vi "FindNodeAtIndex.vi"(8 "ClickIndex":u32=26, 10 "XML with IDs":string="<Sequential ID-O-3=\"\">\n      <Sequential ID-C-1=\"\">\n      </Sequential ID-C-1=\"\">\n      <Drive ID-C-2=\"\"/>\n</Sequential>", 11 "XML In":string="<Sequential>\n      <Sequential>\n      </Sequential>\n      <Drive/>\n</Sequential>") -> (0 "Insert as child not sibling":bool, 1 "Node Name":string="Drive", 3 "Node ID":string)   [LabVIEW 2019]
uses:
  <vilib>/regexp/Match Regular Expression.xnode
panel:
  out "submatch 1":string
  out "String":string
  out "submatch 2":string
  out "Line":i32
  out "Text.Selection:Start":u32=66
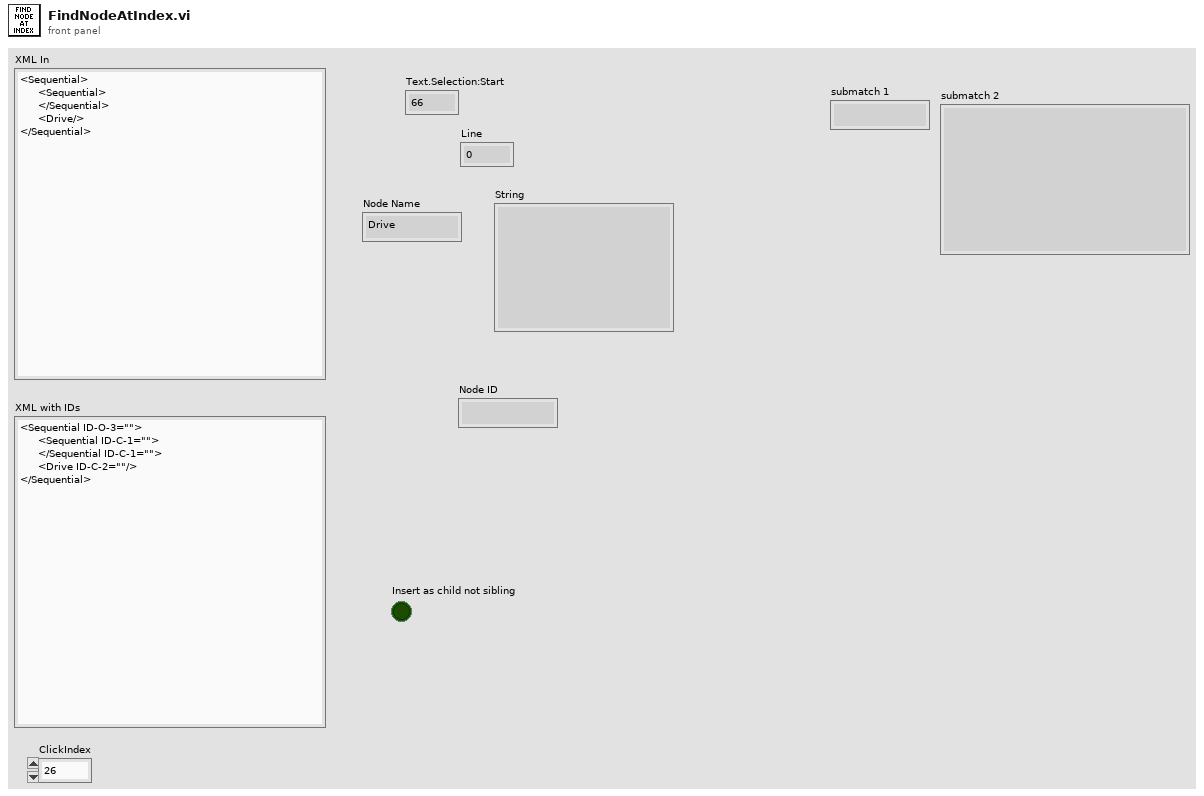
[diagram p1: front panel]
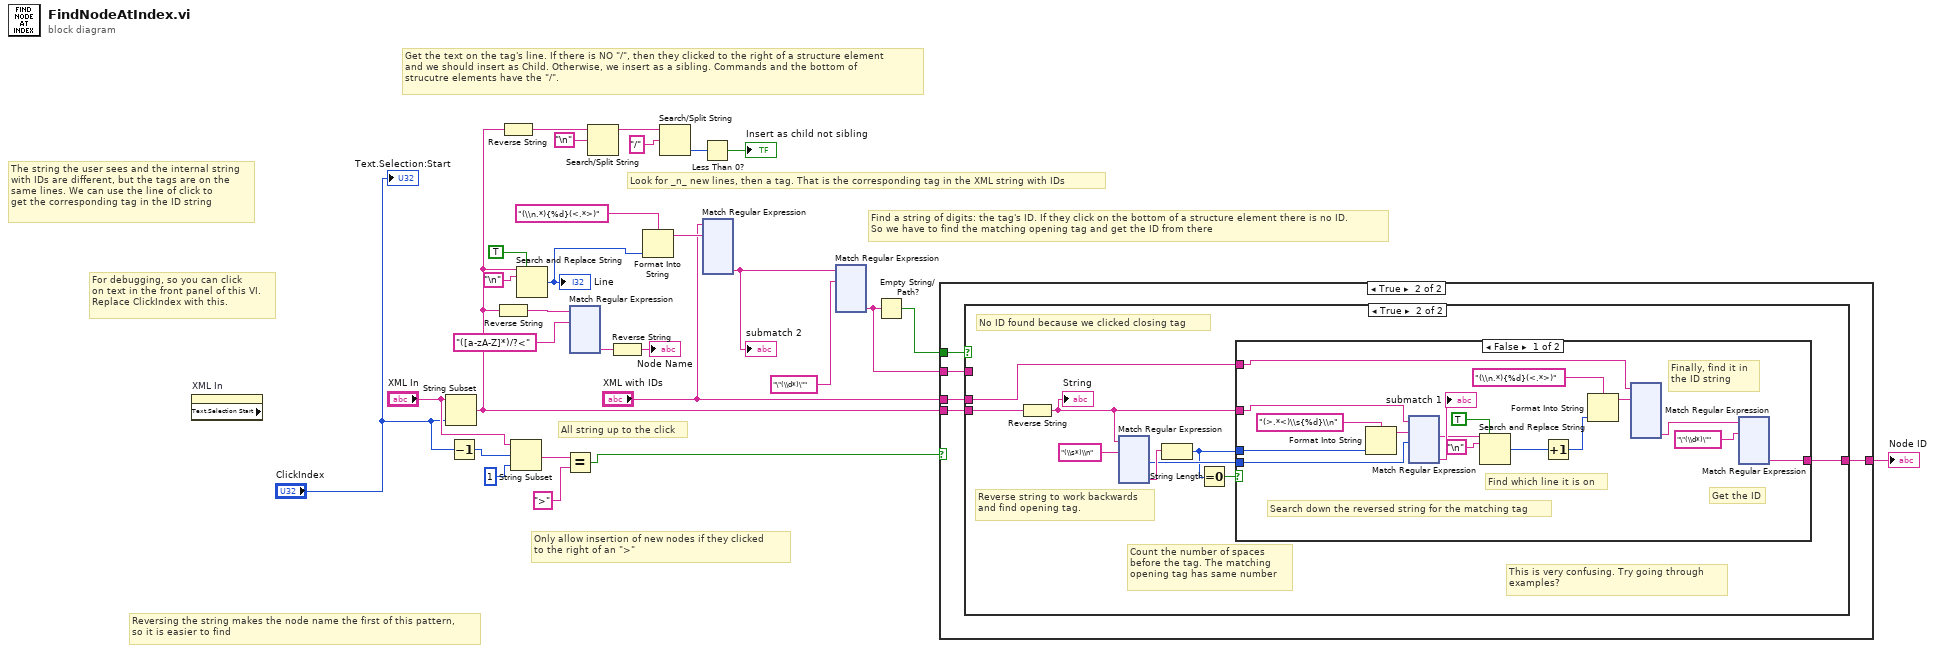
[diagram p0: block diagram]
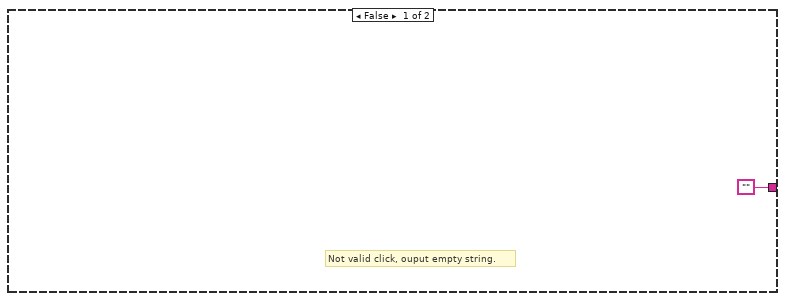
[diagram p2: hidden frame]
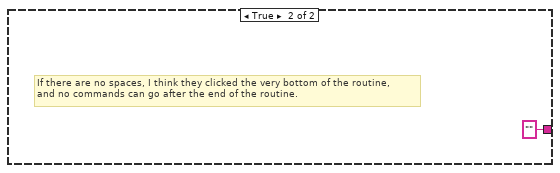
[diagram p4: hidden frame]
diagram:
  # "Find a string of digits: the tag's ID. If they click on the bottom of a structure element there is no ID.\nSo we have to find the matching opening tag and get the ID from there"
  # "Look for _n_ new lines, then a tag. That is the corresponding tag in the XML string with IDs"
  # "Get the text on the tag's line. If there is NO \"/\", then they clicked to the right of a structure element\nand we should insert as Child. Otherwise, we insert as a sibling. Commands and the bottom of\nstrucutre elements have the \"/\"."
  # "The string the user sees and the internal string\nwith IDs are different, but the tags are on the \nsame lines. We can use the line of click to\nget the corresponding tag in the ID string"
  # "Reversing the string makes the node name the first of this pattern,\nso it is easier to find"
  # "All string up to the click"
  # "Only allow insertion of new nodes if they clicked\nto the right of an \">\""
  # "For debugging, so you can click\non text in the front panel of this VI.\nReplace ClickIndex with this."
  n1 = property on="XML In" class="Str" props=["Text", "Selection Start"]() -> ()  [unwired: 2 in, 3 out]
  n2 = String Subset(string="XML In", length (rest)="ClickIndex") -> (substring=w5:string)  [unwired: 1 in]
  n3 = Decrement(x="ClickIndex") -> (x-1=w10:u32)
  n4 = Reverse String(1:w5) -> (0:w4:string)
  n5 = Reverse String(1:w5) -> (0:w28:string)
  n6 = String Subset(string="XML In", offset (0)=w10, length (rest)=1 ("length (rest)")) -> (substring=w8:string)
  n7 = Search and Replace String(replace all?=TRUE ("replace all? (F)"), input string=w5, search string="\n") -> (number of replacements=w19:i32)  [unwired: 5 in, 3 out]
  "Line" <- w19
  n8 = Equal?(x=w8, y=">") -> (x = y?=w6:bool)
  n9 = xnode "Match Regular Expression"("input string"=w4, "regular expression"="([a-zA-Z]*)/?<") -> ("submatch 1"=w3:string)  [unwired: 4 in, 5 out]
  n10 = Search/Split String(string=w28, search string/char (-)="\n") -> (substring before match=w14:string)  [unwired: 1 in, 2 out]
  n11 = Reverse String(1:w3) -> (0:→"Node Name":string)
  n12 = Format Into String(format string="(\\n.*){%d}(<.*>)", w19) -> (resulting string=w20:string)  [unwired: 2 in, 1 out]
  n13 = Search/Split String(string=w14, search string/char (-)="/") -> (offset of match=w29:i32)  [unwired: 1 in, 2 out]
  n14 = Less Than 0?(x=w29) -> (x < 0?=→"Insert as child not sibling":bool)
  n15 = xnode "Match Regular Expression"("input string"="XML with IDs", "regular expression"=w20) -> ("submatch 2"=w18:string)  [unwired: 4 in, 6 out]
  "submatch 2" <- w18
  n16 = xnode "Match Regular Expression"("input string"=w18, "regular expression"="\"(\\d*)\"") -> ("submatch 1"=w15:string)  [unwired: 4 in, 5 out]
  n17 = Empty String/Path?(string/path=w15) -> (empty?=w16:bool)
  n18 = case shown="True" w6 {
    tunnel: w16 -> [_ w35]
    tunnel: w15 -> [_ w34]
    tunnel: w5 -> [_ w33]
    tunnel: ["" w32] -> w13
    tunnel: "XML with IDs" -> [_ w31]
    frame False {
      # "Not valid click, ouput empty string."
    }
    frame True {
      n19 = case shown="True" w35 {
        tunnel: [w36 w40] -> w32
        tunnel: w34 -> [w36 _]
        tunnel: w33 -> [_ w45]
        tunnel: w31 -> [_ w39]
        frame False {
          # "Everything is fine, we know the ID because it was in\nthe tag we clicked and we could easily parse it."
        }
        frame True {
          # "This is very confusing. Try going through\nexamples?"
          # "Reverse string to work backwards\nand find opening tag."
          # "No ID found because we clicked closing tag"
          # "Count the number of spaces\nbefore the tag. The matching\nopening tag has same number"
          n20 = Reverse String(1:w45) -> (0:w42:string)
          "String" <- w42
          n21 = xnode "Match Regular Expression"("input string"=w42, "regular expression"="(\\s*)\\n") -> ("offset past match"=w41:i32, "submatch 1"=w43:string)  [unwired: 4 in, 4 out]
          n22 = String Length(string=w43) -> (length=w38:i32)
          n23 = Equal To 0?(x=w38) -> (x = 0?=w37:bool)
          n24 = case shown="False" w37 {
            tunnel: w42 -> [w62 _]
            tunnel: w41 -> [w61 _]
            tunnel: [w50 "" ("submatch 1")] -> w40
            tunnel: w39 -> [w49 _]
            tunnel: w38 -> [w48 _]
            frame False {
              # "Finally, find it in \nthe ID string"
              # "Find which line it is on"
              # "Get the ID"
              # "Search down the reversed string for the matching tag"
              n25 = Format Into String(format string="(>.*<)\\s{%d}\\n", w48) -> (resulting string=w47:string)  [unwired: 2 in, 1 out]
              n26 = xnode "Match Regular Expression"("input string"=w62, "regular expression"=w47, "offset (0)"=w61) -> ("after match"=w57:string, "submatch 1"=→"submatch 1":string)  [unwired: 3 in, 4 out]
              n27 = Search and Replace String(replace all?=TRUE ("replace all? (F)"), input string=w57, search string="\n") -> (number of replacements=w56:i32)  [unwired: 5 in, 3 out]
              n28 = Increment(x=w56) -> (x+1=w51:i32)
              n29 = Format Into String(format string="(\\n.*){%d}(<.*>)", w51) -> (resulting string=w52:string)  [unwired: 2 in, 1 out]
              n30 = xnode "Match Regular Expression"("input string"=w49, "regular expression"=w52) -> ("submatch 2"=w53:string)  [unwired: 4 in, 6 out]
              n31 = xnode "Match Regular Expression"("input string"=w53, "regular expression"="\"(\\d*)\"") -> ("submatch 1"=w50:string)  [unwired: 4 in, 5 out]
            }
            frame True {
              # "If there are no spaces, I think they clicked the very bottom of the routine,\nand no commands can go after the end of the routine."
            }
          }
        }
      }
    }
  }
  "Node ID" <- w13
  "Text.Selection:Start" <- "ClickIndex"
